vi "Deadband.vi"(7 "Input":dbl) -> (3 "Output":dbl)   [LabVIEW 2018]
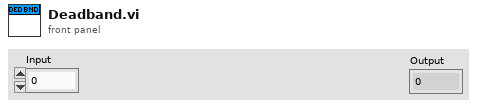
[diagram p1: front panel]
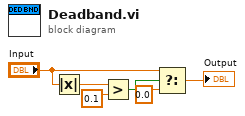
[diagram p0: block diagram]
diagram:
  n1 = Absolute Value(x="Input") -> (abs(x)=w6:dbl)
  n2 = Greater?(x=w6, y=0.1) -> (0:w3:bool)
  n3 = Select(t="Input", s=w3, f=0.0) -> (s? t:f=→"Output":dbl)
